vi "week02_Ex01.vi"() -> ()   [LabVIEW 2017]
panel:
  out "Numeric":i8
  out "x >= y?":bool
  in  "X3":bool
  in  "X2":bool
  in  "X1":bool
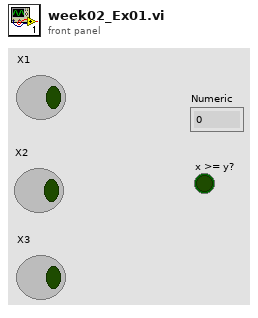
[diagram p1: front panel]
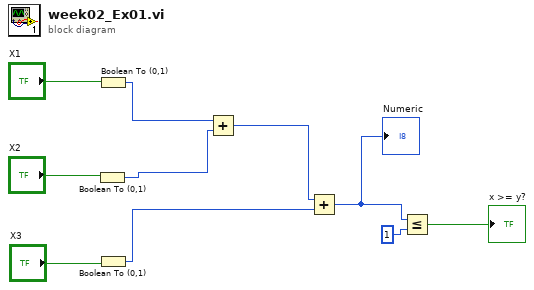
[diagram p0: block diagram]
diagram:
  n1 = Boolean To (0,1)(Boolean="X2") -> (0, 1=w6:i16)
  n2 = Boolean To (0,1)(Boolean="X1") -> (0, 1=w7:i16)
  n3 = Boolean To (0,1)(Boolean="X3") -> (0, 1=w2:i16)
  n4 = Add(x=w7, y=w6) -> (x+y=w5:i16)
  n5 = Add(x=w5, y=w2) -> (x+y=w1:i16)
  "Numeric" <- w1
  n6 = Less Or Equal?(x=w1, y=1) -> (x <= y?=→"x >= y?":bool)
